vi "cv_04-01_arrays.vi"() -> ()   [LabVIEW 2013]
panel:
  out "Reverse Array":dbl[](array[numeric])
  out "Random Array 2":dbl[](array[numeric])
  in  "# of Elements":u32
  in  "Start Subset":u32
  in  "Scaling Factor":dbl
  out "Subset Array":dbl[](array[numeric])
  out "Final Array":dbl[](array[numeric])
  out "Random Array":dbl[](array[numeric])
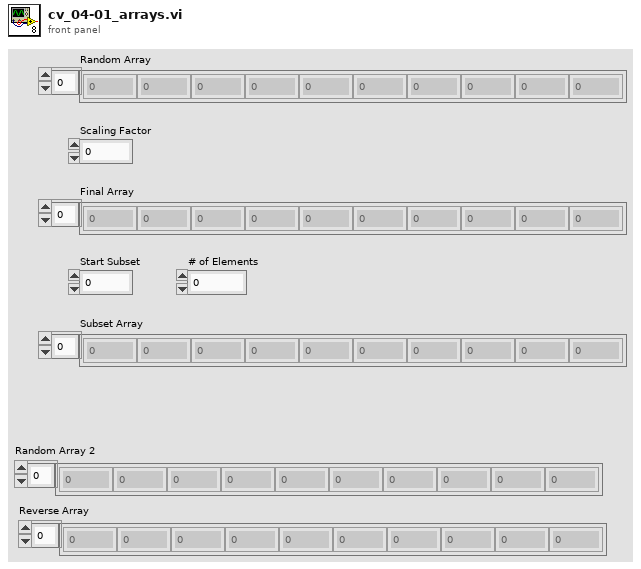
[diagram p1: front panel]
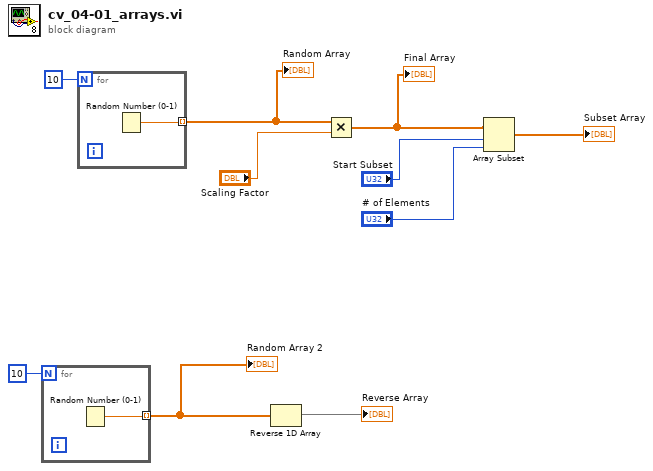
[diagram p0: block diagram]
diagram:
  n1 = for {
    N: 10 -> [_]
    tunnel: [w11] -> w2 mode=indexing
    n2 = Random Number (0-1)() -> (number: 0 to 1=w11:dbl)
  }
  "Random Array 2" <- w2
  n3 = for {
    N: 10 -> [_]
    tunnel: [w12] -> w8 mode=indexing
    n4 = Random Number (0-1)() -> (number: 0 to 1=w12:dbl)
  }
  "Random Array" <- w8
  n5 = Reverse 1D Array(array=w2) -> (reversed array=→"Reverse Array":dbl[])
  n6 = Multiply(x=w8, y="Scaling Factor") -> (x*y=w7:dbl[])
  "Final Array" <- w7
  n7 = Array Subset(array=w7, index="Start Subset", length="# of Elements") -> (→"Subset Array":dbl[])
